vi "CreateSampleMolarMassNode.vi"(8 "Error In":errorcluster, 10 "Sample":T1={"Name"="Sample Name", "Description"="Sample Description", "Molar Mass (g/mol)"=nan, "Density (g/cm^3)"=nan, "Irradiation Area (cm^2)"=nan, "SRIM Damage Peak (disp * ions/cm)"=nan}, 11 "DOM Document In":refnum<k20>) -> (0 "Error out":errorcluster, 2 "Sample Molar Mass Node":refnum<k20>, 3 "DOM Document Out":refnum<k20>)   [LabVIEW 2012]
uses:
  Sample.ctl
  <resource>/objmgr/DOMUserDefRef.rc
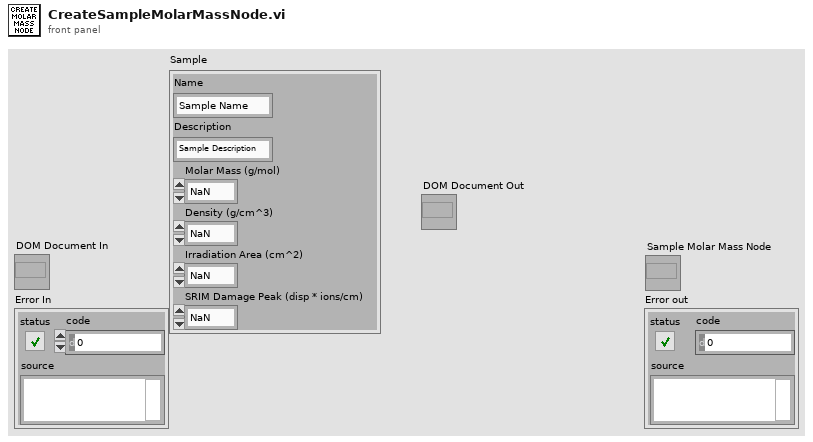
[diagram p1: front panel]
types:
  T1 = typedef "Sample.ctl" = cluster{"Name":string, "Description":string, "Molar Mass (g/mol)":dbl, "Density (g/cm^3)":dbl, "Irradiation Area (cm^2)":dbl, "SRIM Damage Peak (disp * ions/cm)":dbl}
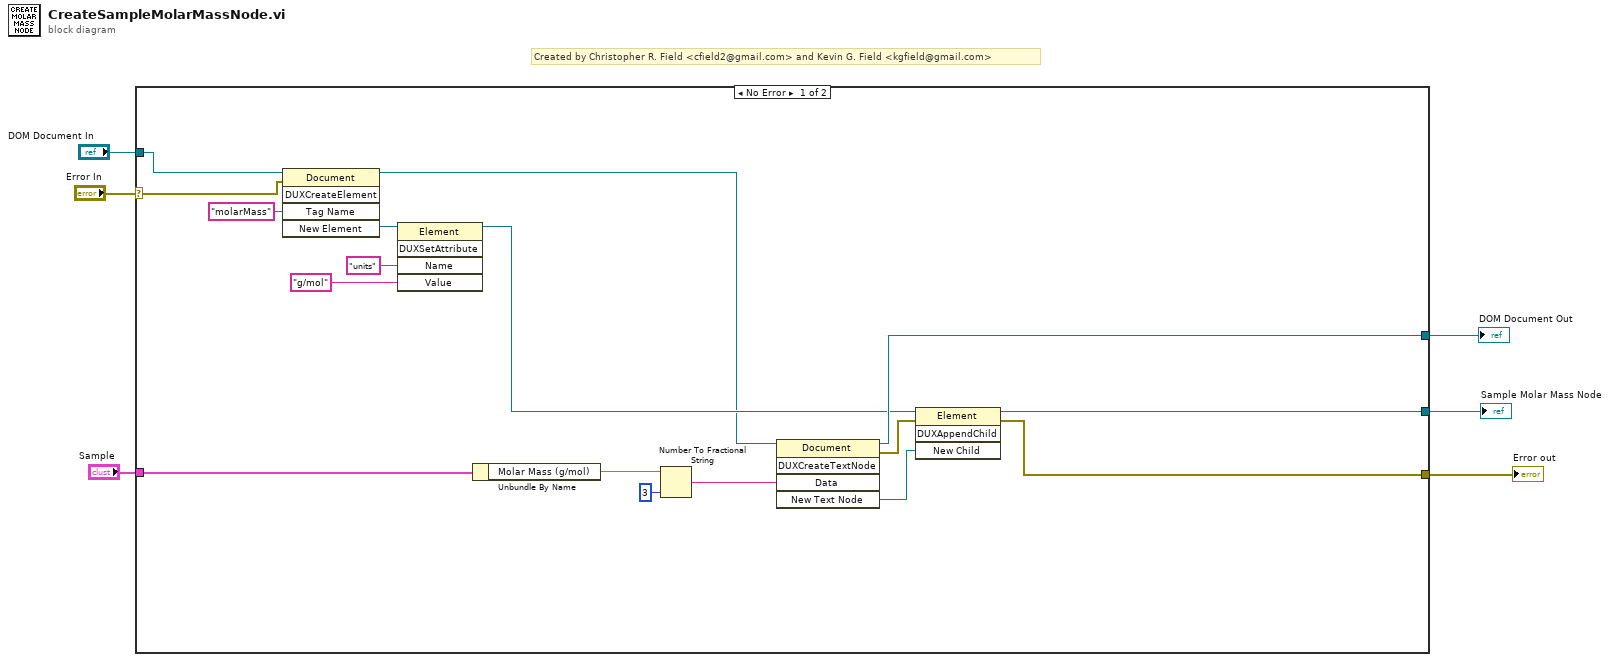
[diagram p0: block diagram]
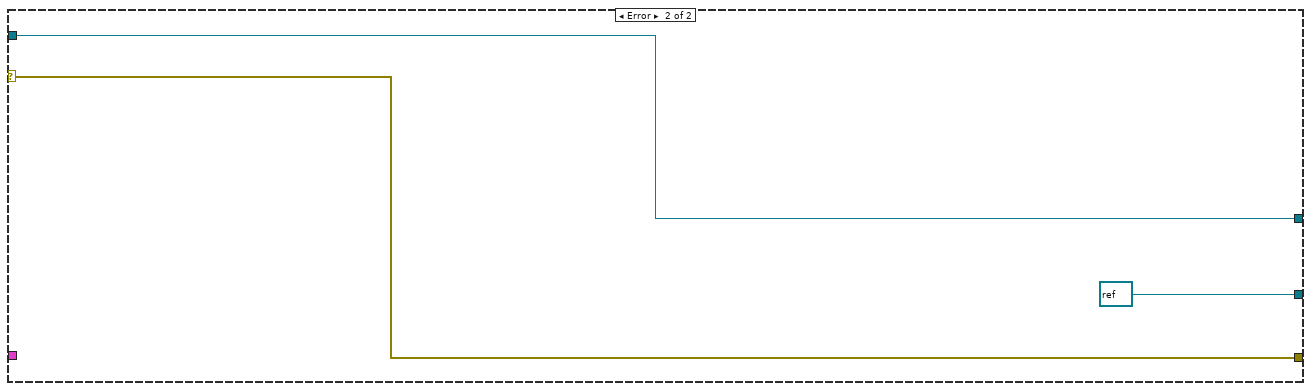
[diagram p2: hidden frame]
diagram:
  # "Created by Christopher R. Field <cfield2@gmail.com> and Kevin G. Field <kgfield@gmail.com>"
  n1 = case shown="No Error" "Error In" {
    selector: "Error In" -> [w16 w25]
    tunnel: "DOM Document In" -> [w23 w26]
    tunnel: [w22 refnum<k20> refnum ("Operator Node 2")] -> w5
    tunnel: [w21 w25] -> w4
    tunnel: "Sample" -> [w17 _]
    tunnel: [w15 w26] -> w2
    frame No Error {
      n2 = invoke class="Document" method="DUXCreateElement"(reference=w23, error in=w16, "Tag Name"="molarMass") -> (reference out=w7:refnum<k20>, "New Element"=w11:refnum<k20>)  [unwired: 2 in, 3 out]
      n3 = invoke class="Element" method="DUXSetAttribute"(reference=w11, "Name"="units", "Value"="g/mol" ("Attribute Value")) -> (reference out=w8:refnum<k20>)  [unwired: 2 in, 4 out]
      n4 = Unbundle By Name(w17) -> ("Molar Mass (g/mol)"=w14:dbl)
      n5 = Number To Fractional String(number=w14, precision (6)=i16 3) -> (F-format string=w12:string)  [unwired: 2 in]
      n6 = invoke class="Document" method="DUXCreateTextNode"(reference=w7, "Data"=w12) -> (reference out=w15:refnum<k20>, error out=w19:errorcluster, "New Text Node"=w18:refnum<k20>)  [unwired: 3 in, 2 out]
      n7 = invoke class="Element" method="DUXAppendChild"(reference=w8, error in=w19, "New Child"=w18) -> (reference out=w22:refnum<k20>, error out=w21:errorcluster)  [unwired: 1 in, 2 out]
    }
    frame Error {
    }
  }
  "Sample Molar Mass Node" <- w5
  "Error out" <- w4
  "DOM Document Out" <- w2
